vi "Get-splitter-references-from-vi.vi"(8 "error in (no error)":errorcluster, 11 "VI Reference":refnum<vi>) -> (0 "error out":errorcluster, 2 "Sorted splitter references":refnum<vi>[](array[refnum]), 3 "VI Reference out":refnum<vi>)   [LabVIEW 2013, in "MaterialCharacterization.lvlib" / "MC-UI.lvclass"]
uses:
  MC-UI.lvclass
  Splitter-names.ctl
  <vilib>/ErrorRing/Error Ring.xnode
panel:
  in  "Splitter-names":T1
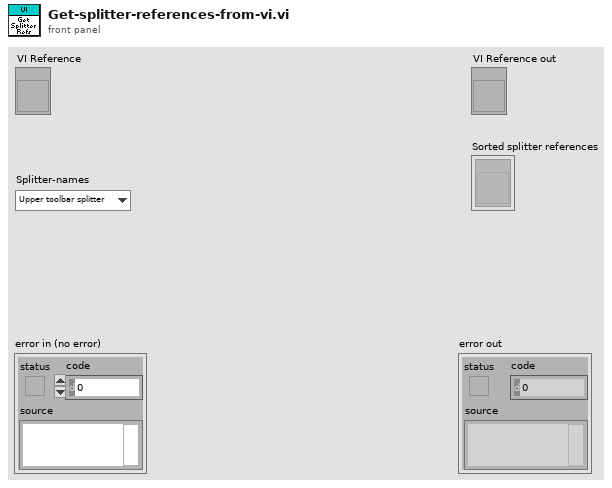
[diagram p1: front panel]
types:
  T1 = typedef "MaterialCharacterization.lvlib/MC-UI.lvclass/Splitter-names.ctl" = enum16{"Upper toolbar splitter", "Help bar splitter", "Lower toolbar splitter", "Upper status bar splitter", "Lower status bar splitter", "Left status bar splitter", "Settings splitter"}
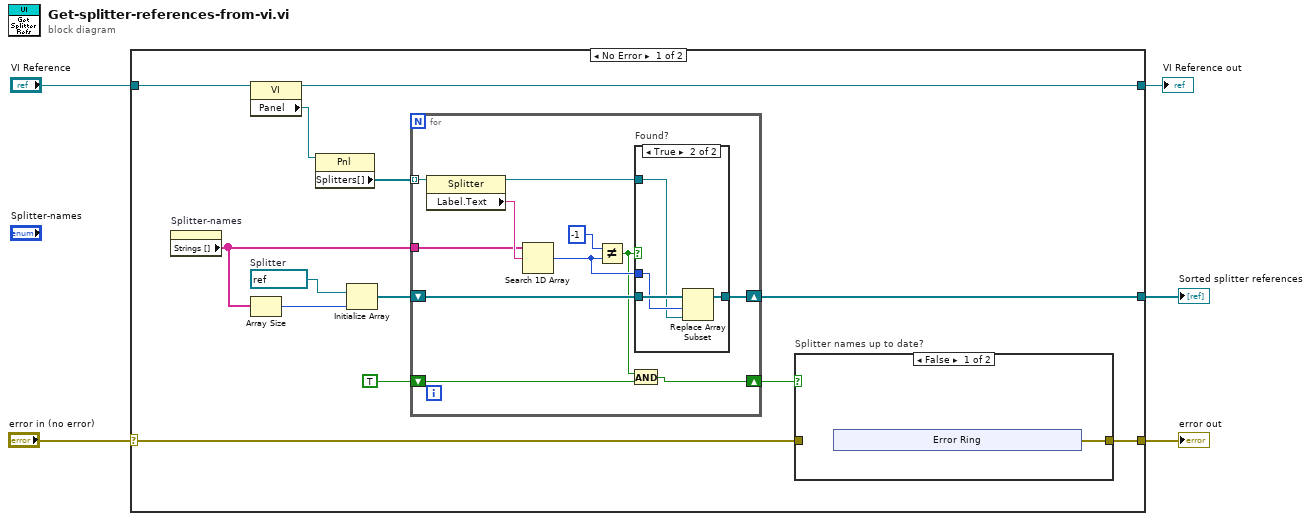
[diagram p0: block diagram]
diagram:
  n1 = case shown="No Error" "error in (no error)" {
    selector: "error in (no error)" -> [w8 w39]
    tunnel: [w7 w39] -> w4
    tunnel: [w12 _] -> w3
    tunnel: "VI Reference" -> [w11 w38]
    tunnel: [w6 w38] -> w1
    frame No Error {
      w13 = refnum<vi> refnum  # Splitter
      n2 = property on="Splitter-names" class="Enum (strict)"() -> ("Strings []"=w14:string[])  [unwired: 2 in, 2 out]
      n3 = property class="VI"(reference=w11) -> (reference out=w6:refnum<vi>, "Panel"=w18:refnum<vi>)  [unwired: 1 in, 1 out]
      n4 = Array Size(array=w14) -> (size(s)=w16:i32)
      n5 = property class="Pnl"(reference=w18) -> ("Splitters[]"=w17:refnum<vi>[])  [unwired: 1 in, 2 out]
      n6 = Initialize Array(w13, w16) -> (w15:refnum<vi>[])
      n7 = for {
        tunnel: w17 -> [w32] mode=indexing
        tunnel: w14 -> [w30]
        shift-right: [w27] -> w12
        shift-left: w15 -> [w28]
        shift-right: [w22] -> w9
        shift-left: TRUE -> [w23]
        n8 = property class="Splitter"(reference=w32) -> (reference out=w26:refnum<vi>, "Label.Text"=w31:string)  [unwired: 1 in, 1 out]
        n9 = Search 1D Array(1D array=w30, element=w31) -> (index of element=w25:i32)  [unwired: 1 in]
        n10 = Not Equal?(x=-1, y=w25) -> (x != y?=w24:bool)
        n11 = And(x=w24, y=w23) -> (x .and. y?=w22:bool)
        n12 = case "Found?" shown="True" w24 {
          tunnel: w28 -> [w33 w37]
          tunnel: [w33 w36] -> w27
          tunnel: w26 -> [_ w34]
          tunnel: w25 -> [_ w35]
          frame False {
          }
          frame True {
            n13 = Replace Array Subset(array=w37, new element=w34, index=w35) -> (w36:refnum<vi>[])
          }
        }
      }
      n14 = case "Splitter names up to date?" shown="False" w9 {
        tunnel: w8 -> [_ w21]
        tunnel: [w19 w21] -> w7
        frame False {
          n15 = xnode "Error Ring"() -> ("error out"=w19:errorcluster)
        }
        frame True {
        }
      }
    }
    frame Error {
    }
  }
  "error out" <- w4
  "Sorted splitter references" <- w3
  "VI Reference out" <- w1
